vi "readMultiple.vi"(0 "refer":refnum<queue>[](array[refnum]), 1 "Index":i32, 2 "wait":bool, 5 "errorIn":errorcluster) -> (11 "remark1":string, 13 "remark 2":string, 14 "refer":refnum<queue>, 15 "to":string, 16 "data":variant, 17 "vaildData":bool, 18 "from":string, 19 "errorOut":errorcluster)   [LabVIEW 2017]
uses:
  models/EMSGData.ctl
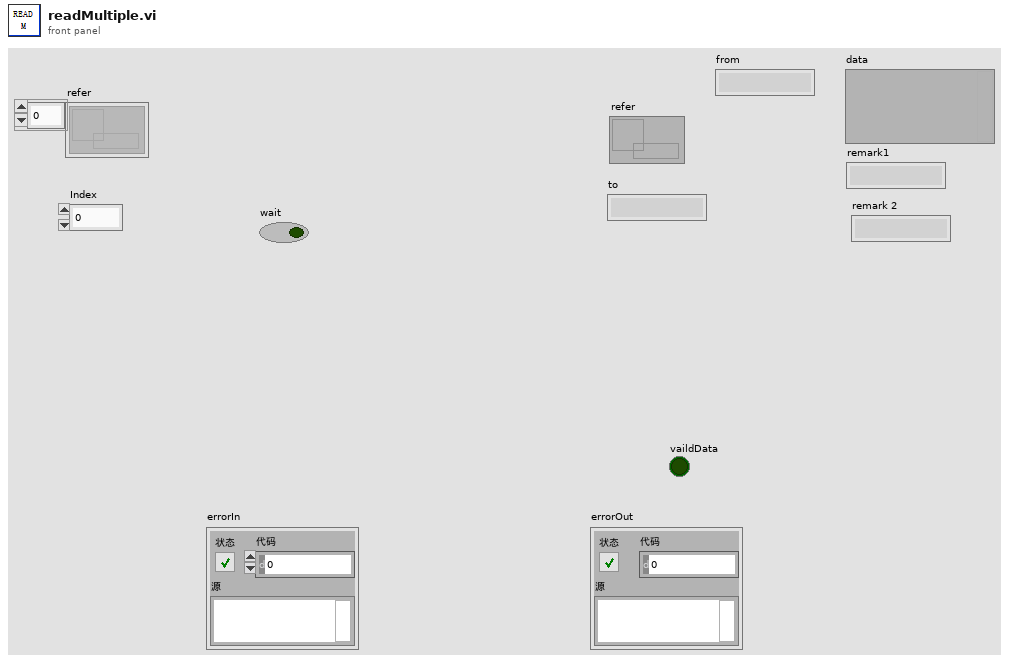
[diagram p1: front panel]
types:
  T1 = typedef "EMSGData.ctl" = cluster{"to":string, "from":string, "data":variant, "remark1":string, "remark 2":string}
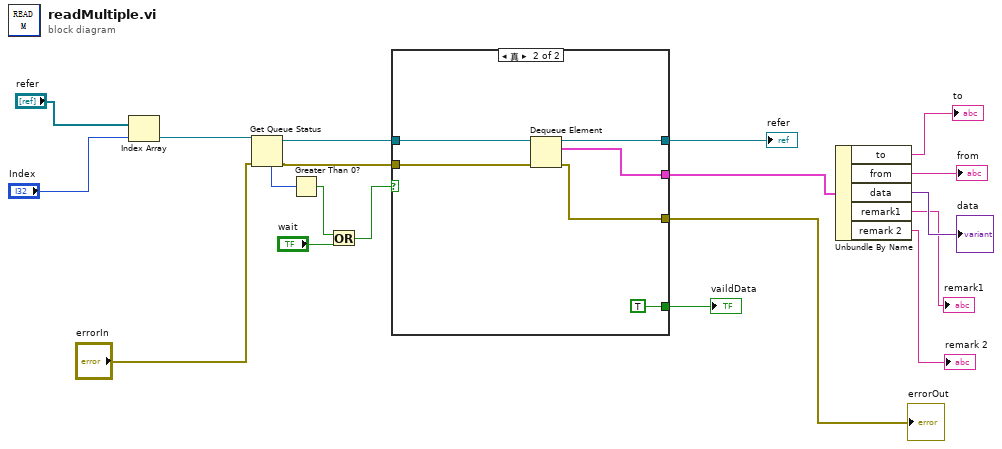
[diagram p0: block diagram]
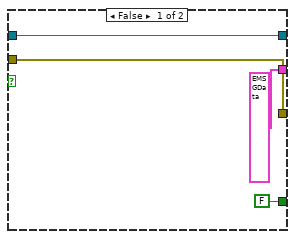
[diagram p2: hidden frame]
diagram:
  n1 = Index Array(array="refer", index="Index") -> (element=w1:refnum<queue>)
  n2 = Get Queue Status(queue=w1, error in (no error)="errorIn") -> (queue out=w18:refnum<queue>, error out=w15:errorcluster, # elements in queue=w17:i32)  [unwired: 1 in, 5 out]
  n3 = Greater Than 0?(x=w17) -> (x > 0?=w13:bool)
  n4 = Or(x=w13, y="wait") -> (x .or. y?=w12:bool)
  n5 = case shown="真" w12 {
    tunnel: [w23 w29] -> w19
    tunnel: [T1 {"to"="", "from"="", "data"=variant, "remark1"="", "remark 2"=""} ("EMSGData") w28] -> w10
    tunnel: [w22 w27] -> w9
    tunnel: w18 -> [w23 w26]
    tunnel: w15 -> [w22 w25]
    tunnel: [FALSE TRUE] -> w11
    frame False {
    }
    frame True {
      n6 = Dequeue Element(queue=w26, error in (no error)=w25) -> (queue out=w29:refnum<queue>, element=w28:T1, error out=w27:errorcluster)  [unwired: 1 in, 1 out]
    }
  }
  "refer" <- w19
  "errorOut" <- w9
  "vaildData" <- w11
  n7 = Unbundle By Name(w10) -> ("to"=→"to":string, "from"=→"from":string, "data"=→"data":variant, "remark1"=→"remark1":string, "remark 2"=→"remark 2":string)
